vi "Read.vi"(1 "Readout parameters":T1(array[cluster]), 3 "Integration time (ms)":u32) -> (0 "Data":dbl[](array[numeric]))   [LabVIEW 2013]
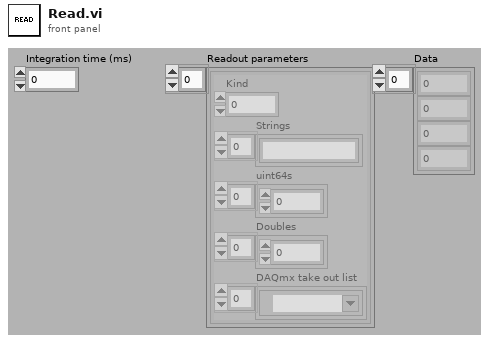
[diagram p1: front panel]
types:
  T1 = cluster{"Kind":u16, "Strings":string[], "uint64s":u64[], "Doubles":dbl[], "DAQmx take out list":refnum<k21>[]}[]
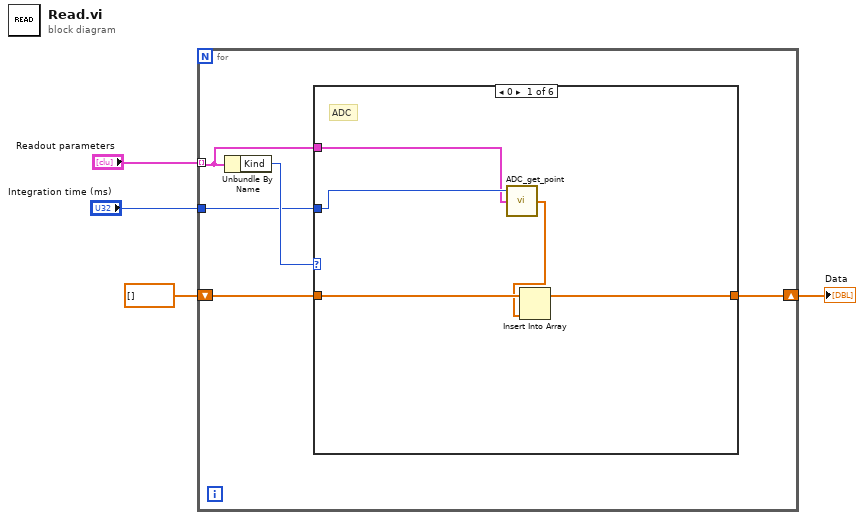
[diagram p0: block diagram]
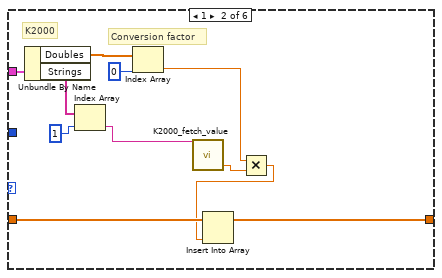
[diagram p2: hidden frame]
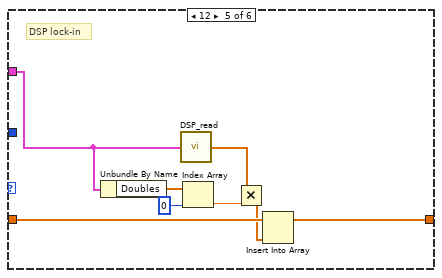
[diagram p5: hidden frame]
diagram:
  n1 = for {
    tunnel: "Readout parameters" -> [w8] mode=indexing
    tunnel: "Integration time (ms)" -> [w7]
    shift-right: [w5] -> w1
    shift-left: dbl[] [] -> [w6]
    n2 = Unbundle By Name(w8) -> ("Kind"=w9:u16)
    n3 = case shown="0" w9 {
      tunnel: w8 -> [w13 w25 _ _ w32 _]
      tunnel: w7 -> [w14 _ _ _ _ _]
      tunnel: w6 -> [w12 w21 w26 w27 w35 w36]
      tunnel: [w11 w20 w26 w27 w34 w36] -> w5
      frame 0 {
        # "ADC"
        n4 = call "ADC_get_point.vi"("Readout parameter"=w13, "Integration time (ms)"=w14) -> ("data"=w10:dbl[])  [unwired: 1 in]
        n5 = Insert Into Array(array=w12, new element=w10) -> (w11:dbl[])  [unwired: 1 in]
      }
      frame 1 {
        # "Conversion factor"
        # "K2000"
        n6 = Unbundle By Name(w25) -> ("Doubles"=w19:dbl[], "Strings"=w23:string[])
        n7 = Index Array(array=w23, index=1) -> (element=w22:string)
        n8 = Index Array(array=w19, index=0) -> (element=w16:dbl)
        n9 = call "K2000_fetch_value.vi"("ResourceNameIn"=w22) -> ("token"=w17:dbl)  [unwired: 1 in, 25 out]
        n10 = Multiply(x=w16, y=w17) -> (x*y=w15:dbl)
        n11 = Insert Into Array(array=w21, new element=w15) -> (w20:dbl[])  [unwired: 1 in]
      }
      frame 2 {
        # "34401A"
      }
      frame 3 {
        # "LeCroy"
      }
      frame 12 {
        # "DSP lock-in"
        n12 = Unbundle By Name(w32) -> ("Doubles"=w31:dbl[])
        n13 = call "DSP_read.vi"("inst param"=w32) -> ("array"=w33:dbl[])
        n14 = Index Array(array=w31, index=0) -> (element=w28:dbl)
        n15 = Multiply(x=w33, y=w28) -> (x*y=w29:dbl[])
        n16 = Insert Into Array(array=w35, new element=w29) -> (w34:dbl[])  [unwired: 1 in]
      }
      frame 100, Default {
        # "If there is no readout instrument,\njst return 0. (It should not happern)"
      }
    }
  }
  "Data" <- w1
